vi "Configure.vi"(0 "SG Path Power Meter Accessor in":refnum<class "SG 2250 Path Accessor.lvclass">, 5 "frequency":dbl=50000000.0, 11 "error in (no error)":errorcluster) -> (4 "SG Path Power Meter Accessor out":refnum<class "SG 2250 Path Accessor.lvclass">, 15 "error out":errorcluster)   [LabVIEW 2023, in "NI-568x RF Power Meter.lvlib" / "SG 2250 Path Accessor.lvclass"]
uses:
  SG 2250 Path Accessor.lvclass
  Power Meter/Power Meter.lvclass
  Power Meter/Power Meter.lvclass/Power Meter.ctl
  Power Meter/Properties/Read Resource Name.vi
  Instruments/Power Meter/Power Meter Factory/Power Meter Factory.lvclass
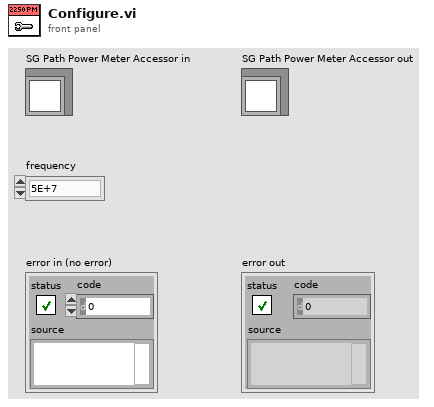
[diagram p1: front panel]
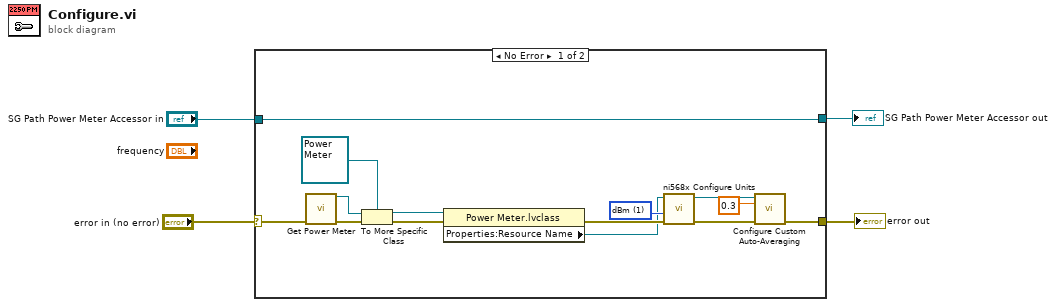
[diagram p0: block diagram]
diagram:
  n1 = case shown="No Error" "error in (no error)" {
    selector: "error in (no error)" -> [w6 w20]
    tunnel: [w18 w20] -> w3
    tunnel: "SG Path Power Meter Accessor in" -> [w5 w19]
    tunnel: [w5 w19] -> w1
    frame No Error {
      w9 = 1 items=["dBm"=1, "Watts"=4, "mWatts"=1001, "uWatts"=1002] ("units")
      n2 = call "Get Power Meter.vi"("error in (no error)"=w6) -> ("Power Meter Base out"=w16:refnum<class "Power Meter Base.lvclass">, "error out"=w15:errorcluster)  [unwired: 13 in]
      n3 = To More Specific Class(target class=refnum<class "Power Meter.lvclass"> refnum ("PM NI568X in"), reference=w16, error in=w15) -> (specific class reference=w13:refnum<class "Power Meter.lvclass">, error out=w14:errorcluster)
      n4 = property class="Power Meter.lvclass"(reference=w13, error in=w14) -> (error out=w8:errorcluster, "Properties:Resource Name"=w7:refnum<k15>)  [unwired: 1 out]
      n5 = call <instrlib>:"ni568x Configure Units.vi"("error in"=w8, "units"=w9, "instrument handle"=w7) -> ("error out"=w10:errorcluster, "instrument handle out"=w11:refnum<k15>)  [unwired: 7 in]
      n6 = call "Configure Custom Auto-Averaging.vi"("reference"=w11, "Initial Aperture Time (s)"=0.3, "error in (no error)"=w10) -> ("error out"=w18:errorcluster)  [unwired: 11 in, 1 out]
    }
    frame Error {
    }
  }
  "error out" <- w3
  "SG Path Power Meter Accessor out" <- w1
